vi "AMZ_S3_Create CanonicalizedAMZHeaders String.vi"(11 "HTTP Headers in":T1[](array[typedef])) -> (2 "CanonicalizedAMZHeaders":string, 3 "HTTP Headers":T1[](array[typedef]))   [LabVIEW 2015, in "LV Interface for Amazon S3.lvlib"]
doc: "Create the CanonicalizedAMZHeaders part of the String to Sign."
uses:
  LV Interface for Amazon S3.lvlib
  Typedefs/AMZ_S3_HTTP Header-Value pair.ctl
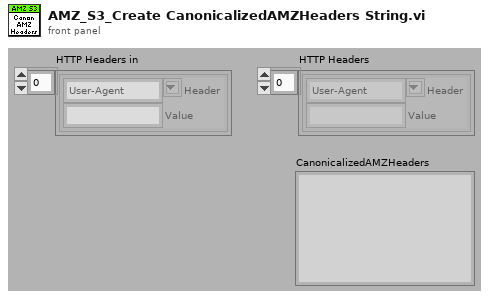
[diagram p1: front panel]
types:
  T1 = typedef "LV Interface for Amazon S3.lvlib/AMZ_S3_HTTP Header-Value pair.ctl" = cluster{"Header":string, "Value":string}
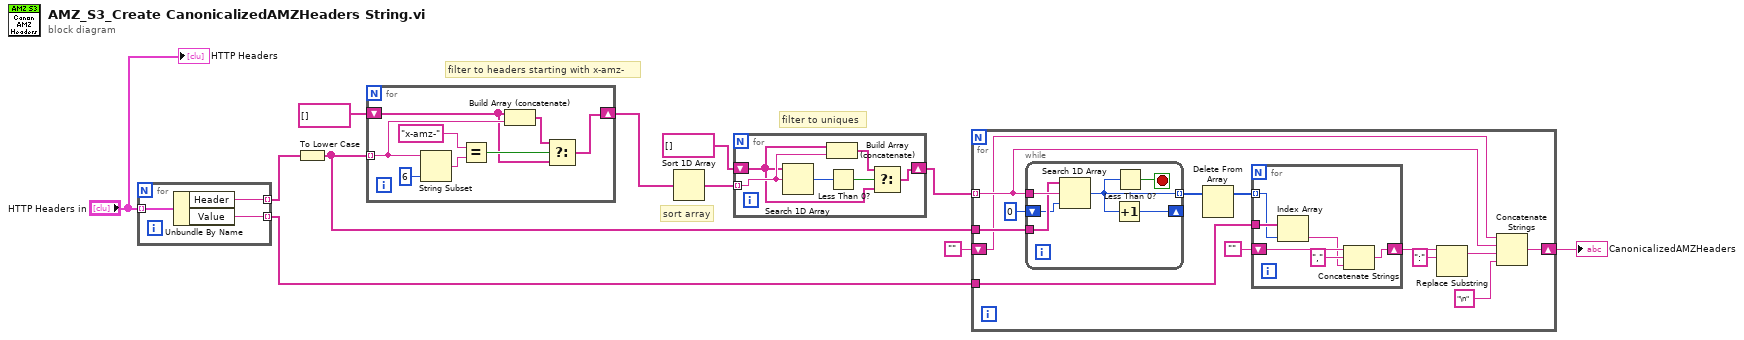
[diagram p0: block diagram]
diagram:
  # "sort array"
  # "filter to headers starting with x-amz-"
  # "filter to uniques"
  n1 = for {
    tunnel: "HTTP Headers in" -> [w14] mode=indexing
    tunnel: [w13] -> w2 mode=indexing
    tunnel: [w12] -> w3 mode=indexing
    n2 = Unbundle By Name(w14) -> ("Header"=w13:string, "Value"=w12:string)
  }
  n3 = To Lower Case(string=w2) -> (all lower case string=w6:string[])
  n4 = for {
    tunnel: w6 -> [w18] mode=indexing
    shift-right: [w16] -> w4
    shift-left: string[] [] -> [w15]
    n5 = String Subset(string=w18, length (rest)=6 ("length (rest)")) -> (substring=w21:string)  [unwired: 1 in]
    n6 = Equal?(x="x-amz-", y=w21) -> (x = y?=w19:bool)
    n7 = Build Array (concatenate)(w15, w18) -> (w17:string[])
    n8 = Select(t=w17, s=w19, f=w15) -> (s? t:f=w16:string[])
  }
  n9 = Sort 1D Array(array=w4) -> (sorted array=w11:string[])
  n10 = for {
    tunnel: w11 -> [w26] mode=indexing
    shift-right: [w23] -> w9
    shift-left: string[] [] -> [w24]
    n11 = Search 1D Array(1D array=w24, element=w26) -> (index of element=w28:i32)  [unwired: 1 in]
    n12 = Build Array (concatenate)(w24, w26) -> (w25:string[])
    n13 = Less Than 0?(x=w28) -> (x < 0?=w27:bool)
    n14 = Select(t=w25, s=w27, f=w24) -> (s? t:f=w23:string[])
  }
  n15 = for {
    tunnel: w9 -> [w33] mode=indexing
    tunnel: w3 -> [w38]
    tunnel: w6 -> [w41]
    shift-right: [w30] -> w7
    shift-left: "" -> [w31]
    n16 = while {
      tunnel: w33 -> [w53]
      tunnel: [w49] -> w40 mode=indexing
      tunnel: w41 -> [w51]
      shift-right: [w48] -> _
      shift-left: 0 -> [w50]
      stop <- w52 stop-if-true
      n17 = Search 1D Array(1D array=w51, element=w53, start index (0)=w50) -> (index of element=w49:i32)
      n18 = Increment(x=w49) -> (x+1=w48:i32)
      n19 = Less Than 0?(x=w49) -> (x < 0?=w52:bool)
    }
    n20 = Delete From Array(array=w40) -> (array with subset deleted=w39:i32[])  [unwired: 2 in, 1 out]
    n21 = for {
      tunnel: w39 -> [w46] mode=indexing
      tunnel: w38 -> [w47]
      shift-right: [w44] -> w36
      shift-left: "" -> [w45]
      n22 = Index Array(array=w47, index=w46) -> (element=w42:string)
      n23 = Concatenate Strings(w45, "," ("string"), w42) -> (w44:string)
    }
    n24 = Replace Substring(4:":" ("substring (\"\")"), 5:w36) -> (1:w34:string)  [unwired: 2 in, 1 out]
    n25 = Concatenate Strings(w31, w33, w34, "\n") -> (w30:string)
  }
  "CanonicalizedAMZHeaders" <- w7
  "HTTP Headers" <- "HTTP Headers in"
